vi "VNA_Display_Sub.vi"(0 "Num points":string="401", 4 "IF Bandwidth":dbl=1000.0, 6 "Span Frequency (MHz)":dbl=50.0, 8 "Center Frequency (GHz)":dbl=10.0, 9 "Trace Format":string(combo)="MLOG", 10 "Measurement Parameter":string(combo)="S21", 11 "VNA Address":refnum<visa-resource-name>="GPIB0::15::INSTR") -> ()   [LabVIEW 2015]
doc: "Display trace from VNA.\nMeasurements parameters: S11, S22, S12, S21\nTrace formats: Linear Magnitude, Logarithmic Magnitude, Phase, Unwrapped Phase, Imaginary, Real, SWR, Group Delay"
panel:
  out "Graph":cluster{dbl[], dbl[]}(graph)
  in  "Stop Now":bool
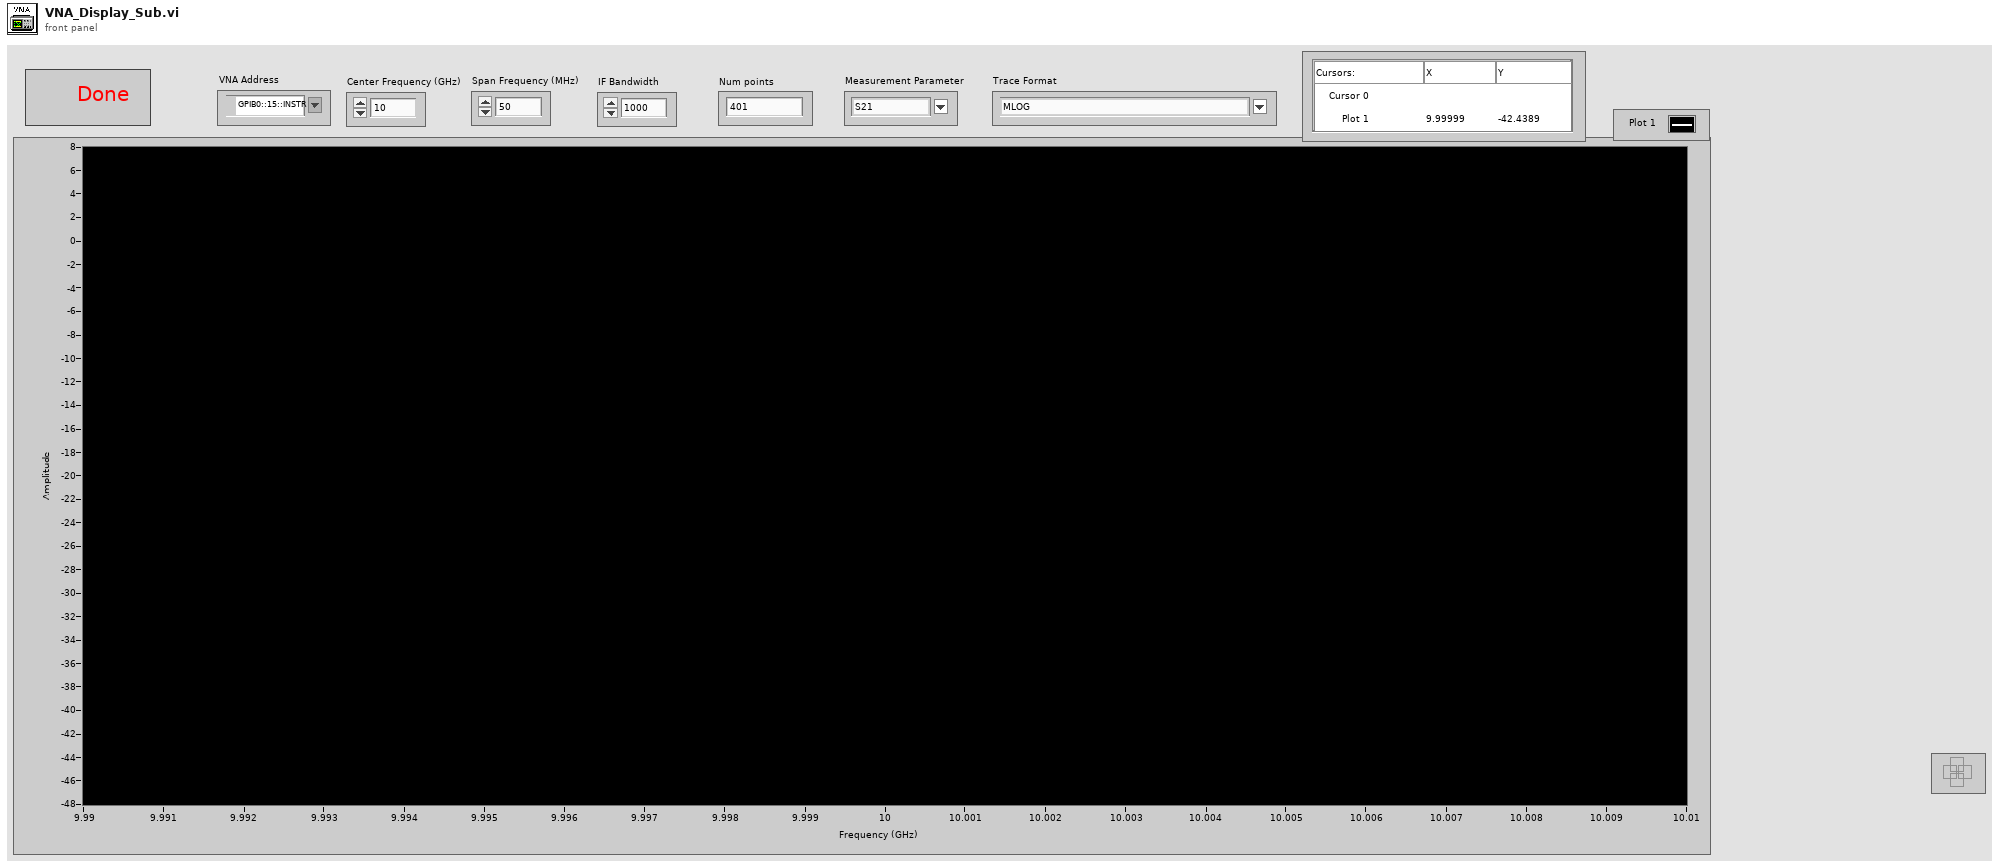
[diagram p1: front panel]
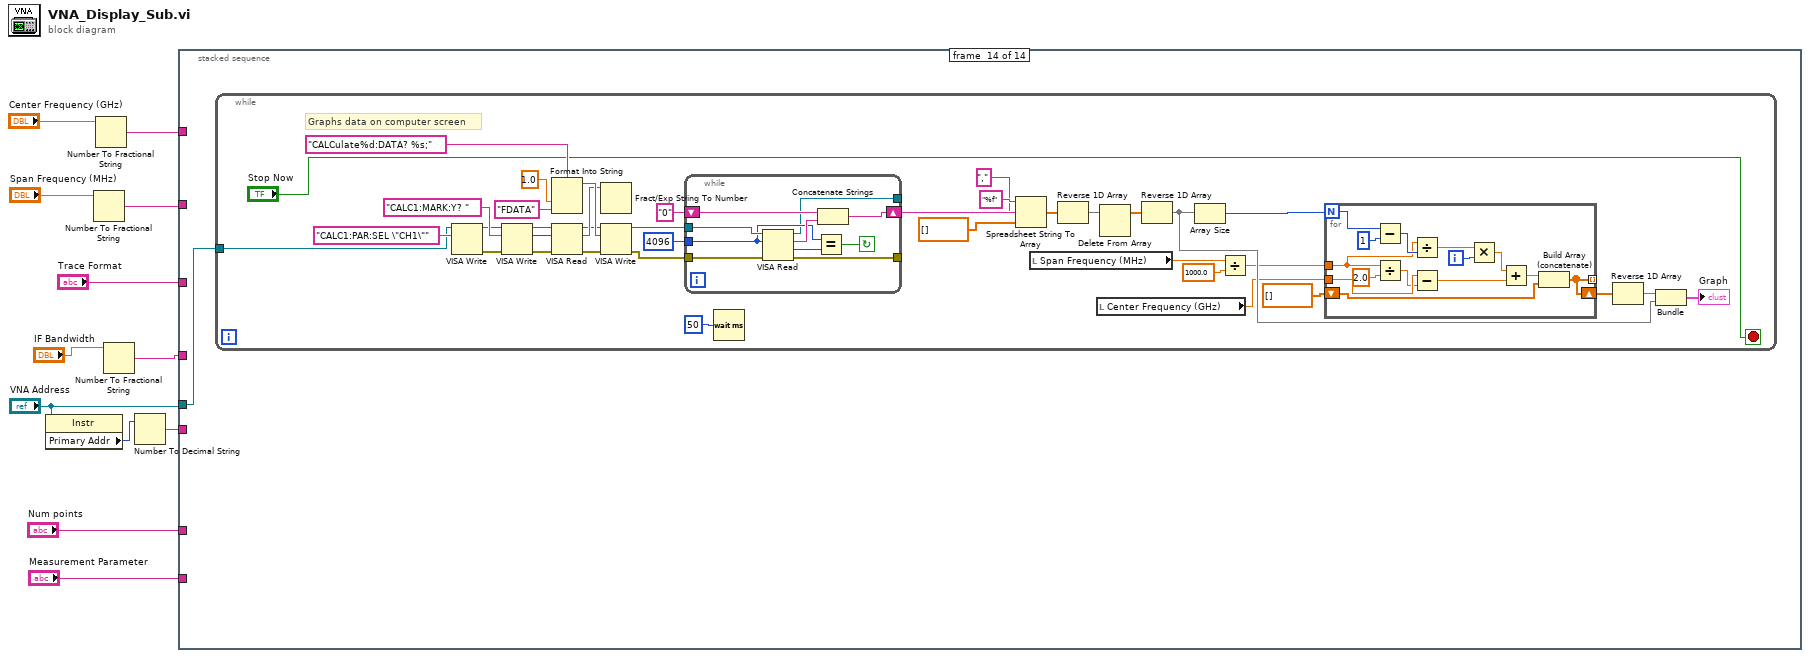
[diagram p0: block diagram]
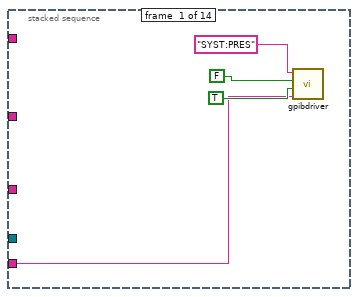
[diagram p2: hidden frame]
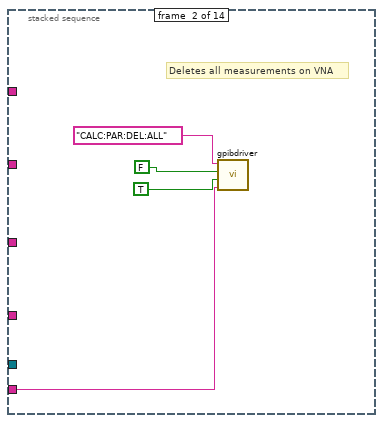
[diagram p3: hidden frame]
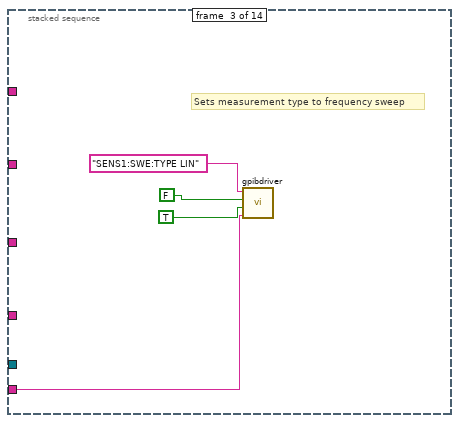
[diagram p4: hidden frame]
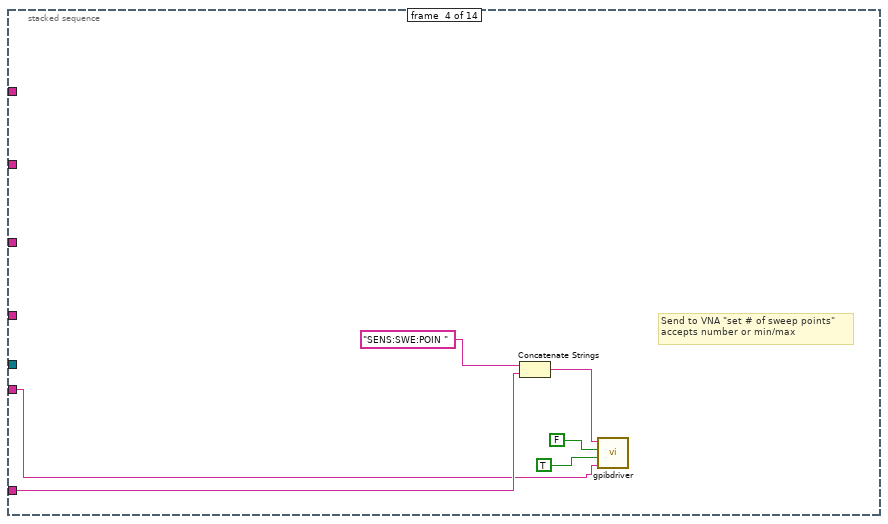
[diagram p5: hidden frame]
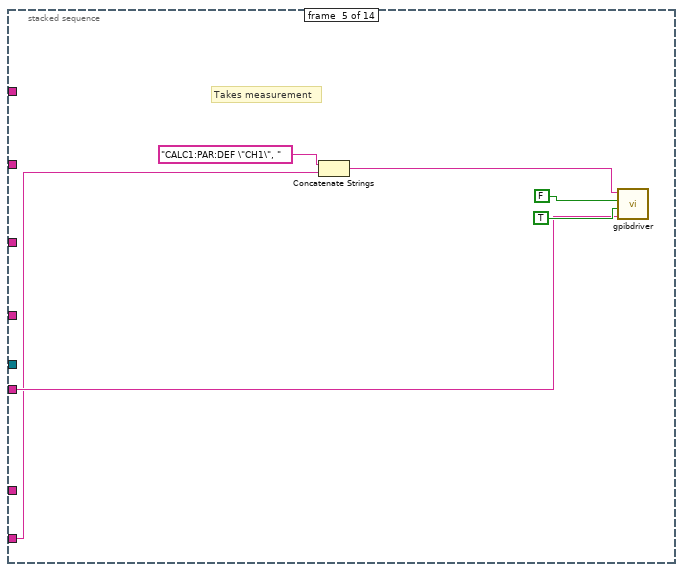
[diagram p6: hidden frame]
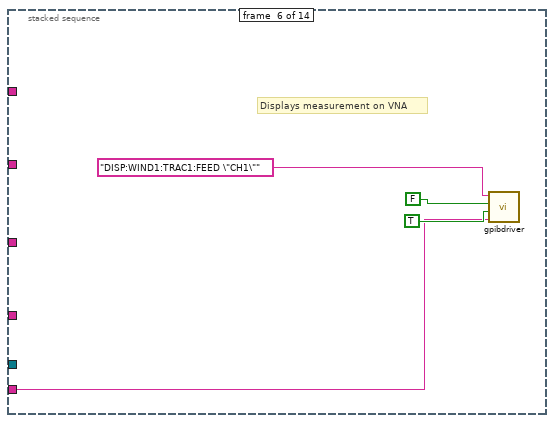
[diagram p7: hidden frame]
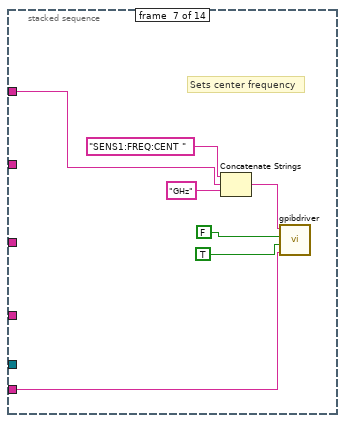
[diagram p8: hidden frame]
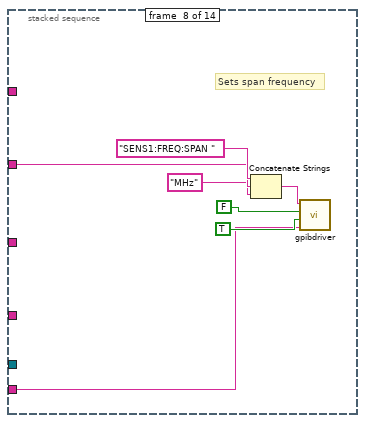
[diagram p9: hidden frame]
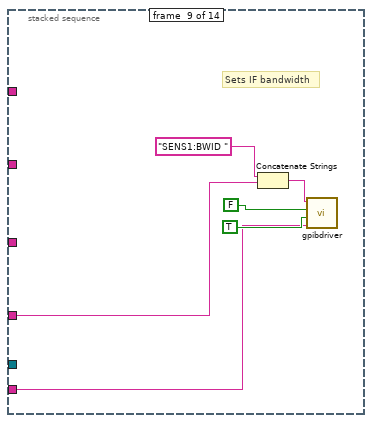
[diagram p10: hidden frame]
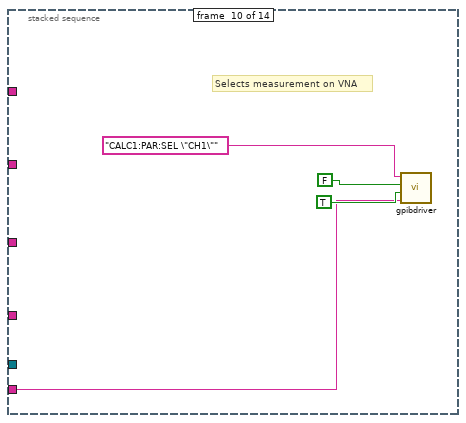
[diagram p11: hidden frame]
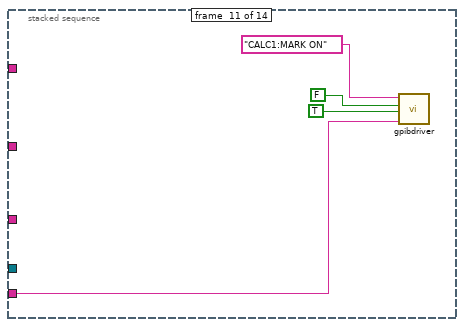
[diagram p12: hidden frame]
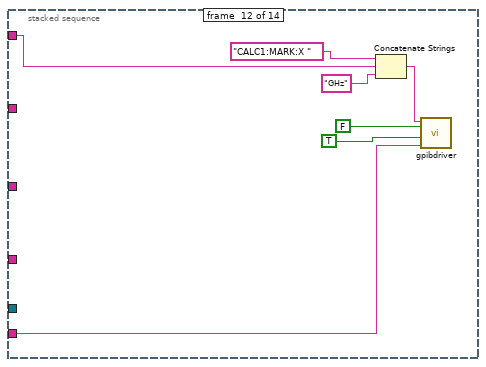
[diagram p13: hidden frame]
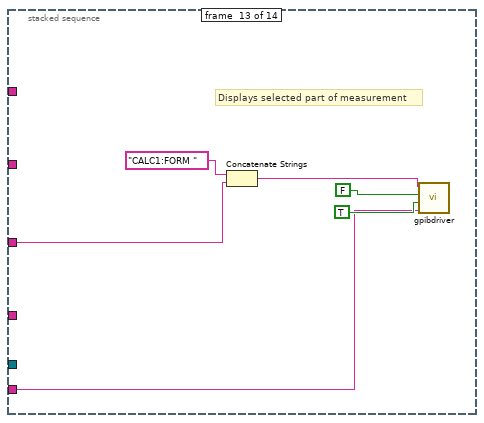
[diagram p14: hidden frame]
diagram:
  n1 = property class="Instr"(reference="VNA Address") -> ("Primary Addr"=w2:u16)  [unwired: 1 in, 2 out]
  n2 = Number To Fractional String(number="Span Frequency (MHz)") -> (F-format string=w11:string)  [unwired: 3 in]
  n3 = Number To Fractional String(number="Center Frequency (GHz)") -> (F-format string=w12:string)  [unwired: 3 in]
  n4 = Number To Fractional String(number="IF Bandwidth") -> (F-format string=w5:string)  [unwired: 3 in]
  n5 = Number To Decimal String(number=w2) -> (decimal integer string=w1:string)  [unwired: 1 in]
  n6 = stacked-sequence {
    tunnel: w5 -> [_ _ _ _ _ _ _ _ w56 _ _ _ _ _]
    tunnel: w1 -> [w13 w17 w21 w25 w34 w38 w42 w49 w55 w62 w65 w71 w79 _]
    tunnel: w12 -> [_ _ _ _ _ _ w44 _ _ _ _ w70 _ _]
    tunnel: w11 -> [_ _ _ _ _ _ _ w50 _ _ _ _ _ _]
    tunnel: "Trace Format" -> [_ _ _ _ _ _ _ _ _ _ _ _ w77 _]
    tunnel: "Measurement Parameter" -> [_ _ _ _ w31 _ _ _ _ _ _ _ _ _]
    tunnel: "Num points" -> [_ _ _ w26 _ _ _ _ _ _ _ _ _ _]
    tunnel: "VNA Address" -> [_ _ _ _ _ _ _ _ _ _ _ _ _ w82]
    frame #0 {
      n7 = call "gpibdriver.vi"("Characters to Write"="SYST:PRES", "Read"=FALSE, "Write"=TRUE ("Write 3"), "GPIB\nAddress"=w13) -> ()  [unwired: 2 in, 1 out]
    }
    frame #1 {
      # "Deletes all measurements on VNA"
      n8 = call "gpibdriver.vi"("Characters to Write"="CALC:PAR:DEL:ALL", "Read"=FALSE, "Write"=TRUE ("Write 3"), "GPIB\nAddress"=w17) -> ()  [unwired: 2 in, 1 out]
    }
    frame #2 {
      # "Sets measurement type to frequency sweep"
      n9 = call "gpibdriver.vi"("Characters to Write"="SENS1:SWE:TYPE LIN", "Read"=FALSE, "Write"=TRUE ("Write 3"), "GPIB\nAddress"=w21) -> ()  [unwired: 2 in, 1 out]
    }
    frame #3 {
      # "Send to VNA \"set # of sweep points\"\naccepts number or min/max"
      n10 = Concatenate Strings("SENS:SWE:POIN " ("Characters to Write"), w26) -> (w27:string)
      n11 = call "gpibdriver.vi"("Characters to Write"=w27, "Read"=FALSE, "Write"=TRUE, "GPIB\nAddress"=w25) -> ()  [unwired: 2 in, 1 out]
    }
    frame #4 {
      # "Takes measurement"
      n12 = Concatenate Strings("CALC1:PAR:DEF \"CH1\", " ("Characters to Write"), w31) -> (w32:string)
      n13 = call "gpibdriver.vi"("Characters to Write"=w32, "Read"=FALSE, "Write"=TRUE ("Write 3"), "GPIB\nAddress"=w34) -> ()  [unwired: 2 in, 1 out]
    }
    frame #5 {
      # "Displays measurement on VNA"
      n14 = call "gpibdriver.vi"("Characters to Write"="DISP:WIND1:TRAC1:FEED \"CH1\"", "Read"=FALSE, "Write"=TRUE ("Write 3"), "GPIB\nAddress"=w38) -> ()  [unwired: 2 in, 1 out]
    }
    frame #6 {
      # "Sets center frequency"
      n15 = Concatenate Strings("SENS1:FREQ:CENT " ("Characters to Write"), w44, "GHz" ("Characters to Write")) -> (w43:string)
      n16 = call "gpibdriver.vi"("Characters to Write"=w43, "Read"=FALSE, "Write"=TRUE ("Write 3"), "GPIB\nAddress"=w42) -> ()  [unwired: 2 in, 1 out]
    }
    frame #7 {
      # "Sets span frequency"
      n17 = Concatenate Strings("SENS1:FREQ:SPAN " ("Characters to Write"), w50, "MHz" ("Characters to Write")) -> (w54:string)
      n18 = call "gpibdriver.vi"("Characters to Write"=w54, "Read"=FALSE, "Write"=TRUE ("Write 3"), "GPIB\nAddress"=w49) -> ()  [unwired: 2 in, 1 out]
    }
    frame #8 {
      # "Sets IF bandwidth"
      n19 = Concatenate Strings("SENS1:BWID " ("Characters to Write"), w56) -> (w60:string)
      n20 = call "gpibdriver.vi"("Characters to Write"=w60, "Read"=FALSE, "Write"=TRUE ("Write 3"), "GPIB\nAddress"=w55) -> ()  [unwired: 2 in, 1 out]
    }
    frame #9 {
      # "Selects measurement on VNA"
      n21 = call "gpibdriver.vi"("Characters to Write"="CALC1:PAR:SEL \"CH1\"", "Read"=FALSE, "Write"=TRUE ("Write 3"), "GPIB\nAddress"=w62) -> ()  [unwired: 2 in, 1 out]
    }
    frame #10 {
      n22 = call "gpibdriver.vi"("Characters to Write"="CALC1:MARK ON", "Read"=FALSE, "Write"=TRUE ("Write 3"), "GPIB\nAddress"=w65) -> ()  [unwired: 2 in, 1 out]
    }
    frame #11 {
      n23 = Concatenate Strings("CALC1:MARK:X " ("Characters to Write"), w70, "GHz" ("string")) -> (w72:string)
      n24 = call "gpibdriver.vi"("Characters to Write"=w72, "Read"=FALSE, "Write"=TRUE ("Write 3"), "GPIB\nAddress"=w71) -> ()  [unwired: 2 in, 1 out]
    }
    frame #12 {
      # "Displays selected part of measurement"
      n25 = Concatenate Strings("CALC1:FORM " ("Characters to Write"), w77) -> (w76:string)
      n26 = call "gpibdriver.vi"("Characters to Write"=w76, "Read"=FALSE, "Write"=TRUE ("Write 3"), "GPIB\nAddress"=w79) -> ()  [unwired: 2 in, 1 out]
    }
    frame #13 {
      n27 = while {
        tunnel: w82 -> [w86]
        stop <- "Stop Now" stop-if-true
        # "Graphs data on computer screen"
        n28 = VISA Write(VISA resource name=w86, write buffer="CALC1:PAR:SEL \"CH1\"" ("Characters to Write")) -> (VISA resource name out=w88:refnum<visa-resource-name>, error out=w89:errorcluster)  [unwired: 1 in, 1 out]
        n29 = VISA Write(VISA resource name=w88, write buffer="CALC1:MARK:Y? " ("Characters to Write"), error in (no error)=w89) -> (VISA resource name out=w93:refnum<visa-resource-name>, return count=w83:u32, error out=w94:errorcluster)
        n30 = Format Into String(format string="CALCulate%d:DATA? %s;", 1.0 ("input 1"), "FDATA") -> (resulting string=w105:string)  [unwired: 2 in, 1 out]
        n31 = VISA Read(VISA resource name=w93, byte count=w83, error in (no error)=w94) -> (VISA resource name out=w85:refnum<visa-resource-name>, read buffer=w92:string, error out=w84:errorcluster)  [unwired: 1 out]
        n32 = Fract/Exp String To Number(string=w92) -> ()  [unwired: 3 in, 2 out]
        n33 = VISA Write(VISA resource name=w85, write buffer=w105, error in (no error)=w84) -> (VISA resource name out=w106:refnum<visa-resource-name>, error out=w95:errorcluster)  [unwired: 1 out]
        n34 = while {
          tunnel: w106 -> [w144]
          tunnel: 4096 -> [w140]
          shift-right: [w142] -> w110
          shift-left: "0" -> [w141]
          tunnel: w95 -> [w137]
          tunnel: [w136] -> _
          tunnel: [w135] -> _
          stop <- w138 continue-if-true
          n35 = VISA Read(VISA resource name=w144, byte count=w140, error in (no error)=w137) -> (VISA resource name out=w135:refnum<visa-resource-name>, read buffer=w143:string, return count=w139:u32, error out=w136:errorcluster)
          n36 = Equal?(x=w140, y=w139) -> (x = y?=w138:bool)
          n37 = Concatenate Strings(w141, w143) -> (w142:string)
        }
        n38 = Wait (ms)(milliseconds to wait=u32 50) -> ()  [unwired: 1 out]
        n39 = Spreadsheet String To Array(delimiter (Tab)=",", format string="%f", spreadsheet string=w110, array type (2D Dbl)=dbl[] []) -> (array=w120:dbl[])
        n40 = local read "Span Frequency (MHz)"() -> (w98:dbl)
        n41 = Reverse 1D Array(array=w120) -> (reversed array=w117:dbl[])
        n42 = local read "Center Frequency (GHz)"() -> (w113:dbl)
        n43 = Delete From Array(array=w117) -> (array with subset deleted=w118:dbl[])  [unwired: 2 in, 1 out]
        n44 = Reverse 1D Array(array=w118) -> (reversed array=w119:dbl[])
        n45 = Array Size(array=w119) -> (size(s)=w114:i32)
        n46 = Divide(x=w98, y=1000.0) -> (x/y=w97:dbl)
        n47 = for {
          N: w114 -> [w134]
          tunnel: w97 -> [w123]
          tunnel: w113 -> [w125]
          shift-right: [w126] -> w115
          shift-left: dbl[] [] -> [w127]
          tunnel: [w126] -> _ mode=indexing
          i -> [w130]
          n48 = Subtract(x=w134, y=1 ("x+y")) -> (x-y=w132:i32)
          n49 = Divide(x=w123, y=2.0) -> (x/y=w124:dbl)
          n50 = Divide(x=w123, y=w132) -> (x/y=w131:dbl)
          n51 = Subtract(x=w125, y=w124) -> (x-y=w121:dbl)
          n52 = Multiply(x=w131, y=w130) -> (x*y=w129:dbl)
          n53 = Add(x=w129, y=w121) -> (x+y=w128:dbl)
          n54 = Build Array (concatenate)(w128, w127) -> (w126:dbl[])
        }
        n55 = Reverse 1D Array(array=w115) -> (reversed array=w101:dbl[])
        n56 = Bundle(w101, w119) -> (→"Graph":cluster{dbl[], dbl[]})  [unwired: 1 in]
      }
    }
  }
